vi "Colors Construct.vi"() -> ()   [LabVIEW 2015]
uses:
  Controls/Ti Colors.ctl
panel:
  out "output array 2":u32[](array[colorbox])
  out "unsigned 32bit integer":u32
  in  "stop":bool
  out "output array":u32[][](array[colorbox])
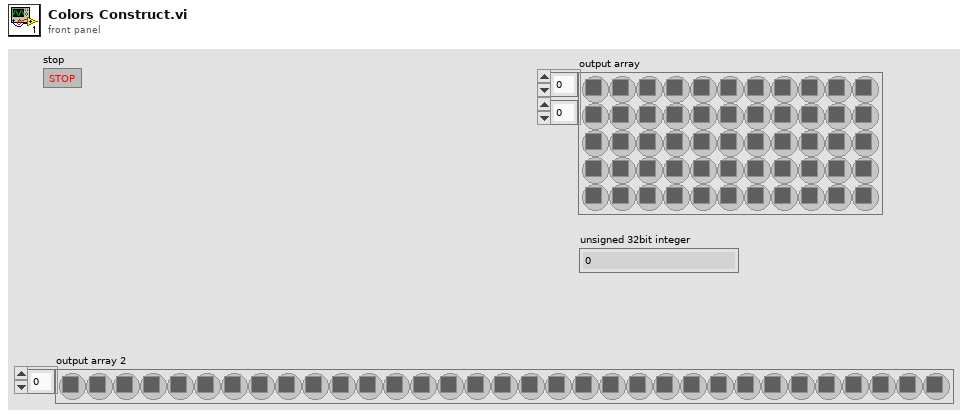
[diagram p1: front panel]
types:
  T1 = typedef "Ti Colors.ctl" = u32[]
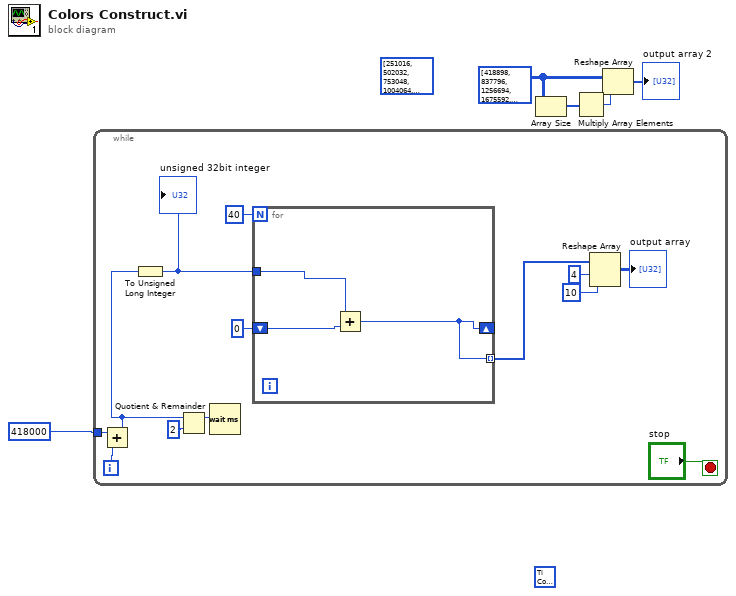
[diagram p0: block diagram]
diagram:
  (unwired) T1 [418898, 837796, 1256694, 1675592, 2094490, 2513388, 2932286, 3351184, 3770082, 4188980, 4607878, 5026776, 5445674, 5864572, 6283470, 6702368, 7121266, 7540164, 7959062, 8377960, 8796858, 9215756, 9634654, 10053552, 10472450, 10891348, 11310246, 11729144, 12148042, 12566940, 12985838, 13404736, 13823634, 14242532, 14661430, 15080328, 15499226, 15918124, 16337022, 16755920] ("output array 2")
  w3 = u32[][] [[418898, 837796, 1256694, 1675592, 2094490, 2513388, 2932286, 3351184, 3770082, 4188980], [4607878, 5026776, 5445674, 5864572, 6283470, 6702368, 7121266, 7540164, 7959062, 8377960], [8796858, 9215756, 9634654, 10053552, 10472450, 10891348, 11310246, 11729144, 12148042, 12566940], [12985838, 13404736, 13823634, 14242532, 14661430, 15080328, 15499226, 15918124, 16337022, 16755920]] ("output array")
  (unwired) u32[][] [[251016, 502032, 753048, 1004064, 1255080, 1506096, 1757112, 2008128, 2259144, 2510160], [2761176, 3012192, 3263208, 3514224, 3765240, 4016256, 4267272, 4518288, 4769304, 5020320], [5271336, 5522352, 5773368, 6024384, 6275400, 6526416, 6777432, 7028448, 7279464, 7530480], [7781496, 8032512, 8283528, 8534544, 8785560, 9036576, 9287592, 9538608, 9789624, 10040640]] ("output array 2")
  n1 = while {
    tunnel: 418000 -> [w6]
    i -> [w10]
    stop <- "stop" stop-if-true
    n2 = Add(x=w6, y=w10) -> (x+y=w7:i32)
    n3 = To Unsigned Long Integer(number=w7) -> (unsigned 32bit integer=w11:u32)
    "unsigned 32bit integer" <- w11
    n4 = Quotient & Remainder(x=w7, y=2) -> (x-y*floor(x/y)=w8:i32)  [unwired: 1 out]
    n5 = Wait (ms)(milliseconds to wait=w8) -> ()  [unwired: 1 out]
    n6 = for {
      N: 40 -> [_]
      tunnel: [w20] -> w17 mode=indexing
      shift-right: [w20] -> _
      shift-left: u32 0 -> [w21]
      tunnel: w11 -> [w19]
      n7 = Add(x=w19, y=w21) -> (x+y=w20:u32)
    }
    n8 = Reshape Array(w17, 4 ("dimension size"), 10 ("dimension size")) -> (→"output array":u32[][])
  }
  n9 = Array Size(array=w3) -> (size(s)=w2:i32[])
  n10 = Multiply Array Elements(1:w2) -> (0:w1:i32)
  n11 = Reshape Array(w3, w1) -> (→"output array 2":u32[])
